vi "Write SAL_Library.vi"(8 "error in (no error)":errorcluster, 10 "SAL_Library":string, 11 "ProgrammaticInitialization in":refnum<class "ProgrammaticInitialization.lvclass">) -> (0 "error out":errorcluster, 3 "ProgrammaticInitialization out":refnum<class "ProgrammaticInitialization.lvclass">)   [LabVIEW 2016, in "ProgrammaticInitialization.lvclass"]
uses:
  ProgrammaticInitialization.lvclass
  ProgrammaticInitialization.lvclass/ProgrammaticInitialization.ctl
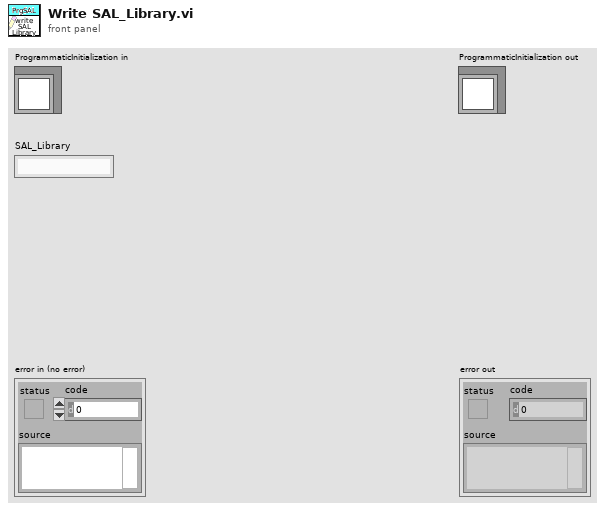
[diagram p1: front panel]
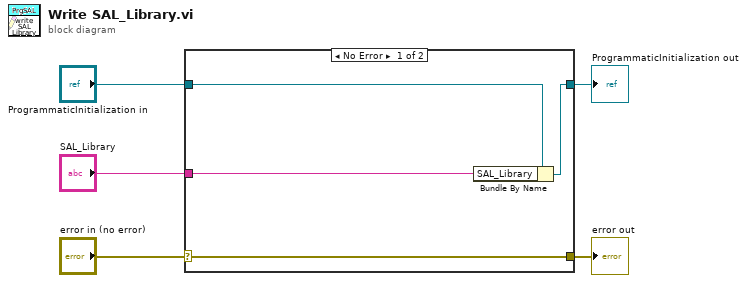
[diagram p0: block diagram]
diagram:
  n1 = case shown="No Error" "error in (no error)" {
    selector: "error in (no error)" -> [w9 w10]
    tunnel: [w9 w10] -> w4
    tunnel: [w7 w11] -> w2
    tunnel: "ProgrammaticInitialization in" -> [w8 w11]
    tunnel: "SAL_Library" -> [w6 _]
    frame No Error {
      n2 = Bundle By Name(cluster=w8, "SAL_Library"=w6) -> (w7:refnum<class "ProgrammaticInitialization.lvclass">)
    }
    frame Error {
    }
  }
  "error out" <- w4
  "ProgrammaticInitialization out" <- w2
